vi "test7.vi"   [LabVIEW 2012]
uses:
  <vilib>/NXT/Subs/MotorOutput.ctl
  <vilib>/NXT/Block Support/NXT_InputPort.ctl
  <vilib>/NXT/Dual Mode Library/Motors/MotorOn.vi
  <vilib>/NXT/Dual Mode Library/Motors/MotorBrake.vi
  <vilib>/NXT/Dual Mode Library/Display/drawNumber.vi
  <vilib>/NXT/Dual Mode Library/Waits/Wait_Num.vi
  <vilib>/NXT/Dual Mode Library/Waits/Wait_Num(msec).vi
  <vilib>/NXT/Dual Mode Library/Display/drawLine.vi
types:
  T1 = typedef "MotorOutput.ctl" = u8
  T2 = typedef "LVHSConnector.ctl" = cluster{"Hardware":string, "Flattened String":string}
  T3 = typedef "NXT_InputPort.ctl" = u8
  T4 = cluster{"x-y*floor(x/y)":i32, "Start X":i16, "x-y*floor(x/y)":i32, i8}
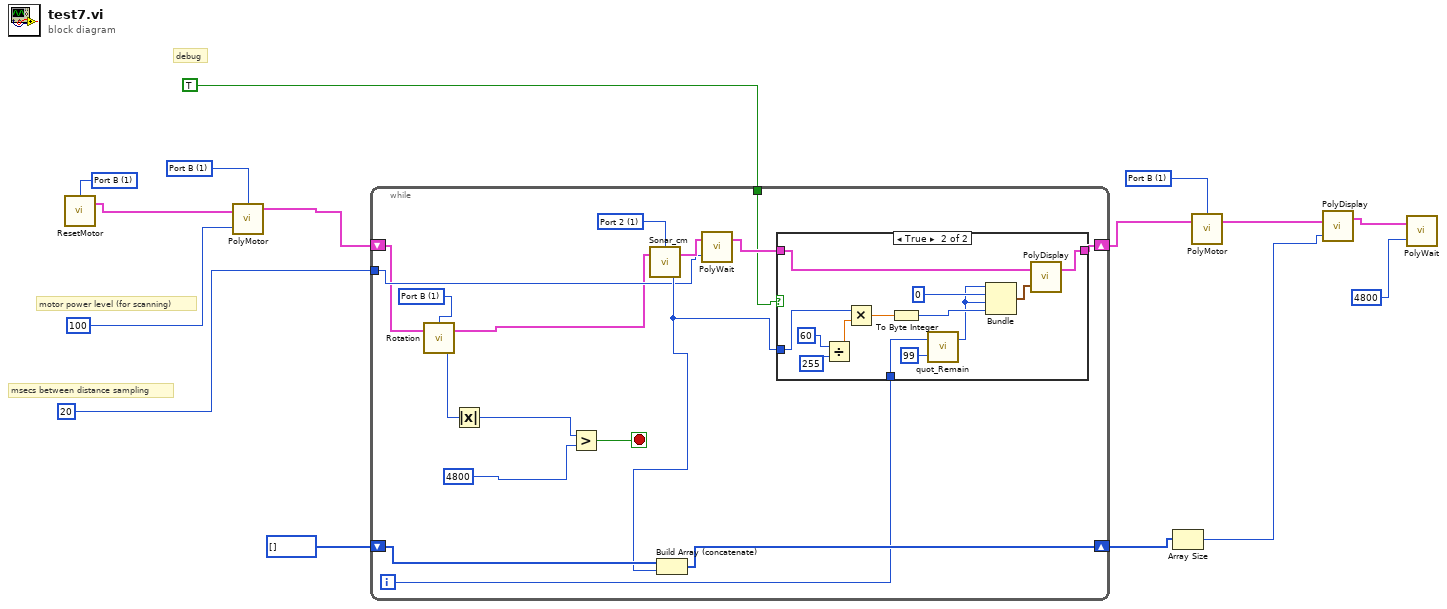
[diagram p0: block diagram]
diagram:
  w8 = T1 1 items=["Port A"=0, "Port B"=1, "Port C"=2, "Ports A & B"=4, "Ports A & C"=5, "Ports B & C"=6, "as"=3] ("Output Port (All Ports)")
  w10 = T1 1 items=["Port A"=0, "Port B"=1, "Port C"=2, "Ports A & B"=4, "Ports A & C"=5, "Ports B & C"=6, "All Ports"=3] ("Port (All Ports)")
  w15 = T1 1 items=["Port A"=0, "Port B"=1, "Port C"=2, "Ports A & B"=4, "Ports A & C"=5, "Ports B & C"=6, "as"=3] ("Output Port (All Ports)")
  # "msecs between distance sampling"
  # "motor power level (for scanning)"
  # "debug"
  n1 = call <vilib>:"ResetMotor.vi"("Port (All Ports)"=w10) -> ("NXT"=w9:T2)  [unwired: 3 in]
  n2 = call-poly <vilib>:"PolyMotor.vi"("Power (75)"=100, "NXT"=w9, "Output Port (All Ports)"=w15) -> ("NXT"=w6:T2)  [unwired: 1 in]
  n3 = while {
    shift-right: [w30] -> w4
    shift-left: i16[] [] -> [w31]
    tunnel: TRUE -> [w26]
    tunnel: 20 -> [w23]
    shift-right: [w27] -> w7
    shift-left: w6 -> [w19]
    i -> [w24]
    stop <- w20 stop-if-true
    w22 = T1 1 items=["Port A"=0, "Port B"=1, "Port C"=2, "Ports A & B"=4, "Ports A & C"=5, "Ports B & C"=6, "as"=3] ("Output Port (All Ports)")
    w32 = T3 1 items=["Port 1", "Port 2", "Port 3", "Port 4"] ("Port (Port 4)")
    n4 = call <vilib>:"Rotation.vi"("NXT"=w19, "Port (Port A)"=w22) -> ("Angle of Rotation"=w21:i32, "NXT"=w18:T2)  [unwired: 1 in]
    n5 = Absolute Value(x=w21) -> (abs(x)=w17:i32)
    n6 = Greater?(x=w17, y=i16 4800 ("Max Value")) -> (0:w20:bool)
    n7 = call <vilib>:"Sonar_cm.vi"("NXT"=w18, "Port (Port 4)"=w32) -> ("Distance (cm)"=w25:i16, "NXT"=w29:T2)  [unwired: 1 in]
    n8 = Build Array (concatenate)(w31, w25) -> (w30:i16[])
    n9 = call-poly <vilib>:"PolyWait.vi"("Time (100 msec)"=w23, "NXT"=w29) -> ("NXT"=w28:T2)  [unwired: 2 in]
    n10 = case shown="True" w26 {
      tunnel: w28 -> [w33 w43]
      tunnel: [w33 w44] -> w27
      tunnel: w25 -> [_ w42]
      tunnel: w24 -> [_ w35]
      frame False {
      }
      frame True {
        n11 = Divide(x=i16 60 ("Start X"), y=i16 255 ("Start X")) -> (x/y=w40:dbl)
        n12 = Multiply(x=w42, y=w40) -> (x*y=w45:dbl)
        n13 = To Byte Integer(number=w45) -> (8bit integer=w37:i8)
        n14 = call <vilib>:"quot_Remain.vi"("y"=i16 99 ("Start X"), "x"=w35) -> ("x-y*floor(x/y)"=w36:i32)  [unwired: 1 out]
        n15 = Bundle("x-y*floor(x/y)"=w36, "Start X"=i16 0, "x-y*floor(x/y)"=w36, w37) -> (w38:T4)  [unwired: 1 in]
        n16 = call-poly <vilib>:"PolyDisplay.vi"("Line Parameters"=w38, "NXT"=w43) -> ("NXT"=w44:T2)  [unwired: 2 in]
      }
    }
  }
  n17 = Array Size(array=w4) -> (size(s)=w3:i32)
  n18 = call-poly <vilib>:"PolyMotor.vi"("NXT"=w7, "Port (All Ports)"=w8) -> ("NXT"=w5:T2)  [unwired: 2 in]
  n19 = call-poly <vilib>:"PolyDisplay.vi"("number"=w3, "NXT"=w5) -> ("NXT"=w2:T2)  [unwired: 2 in]
  n20 = call-poly <vilib>:"PolyWait.vi"("Time (1 sec)"=i16 4800 ("Max Value"), "NXT"=w2) -> ()  [unwired: 2 in, 1 out]
